vi "Event Start On Track.vi"(6 "Track ID":u64, 7 "Event Name":string, 8 "error in":errorcluster) -> (0 "error out":errorcluster)   [LabVIEW 2027, in "VS Tracing API.lvlib"]
doc: "Records the start of a user-space event on a previously registered custom track. The event remains active until the corresponding <i>Event Stop On Track</i> is called.\nUse this VI when recording events outside timed structures or when events need to be associated with a specific custom track.\n\n<b>Parameters</b>\n• <b>Track ID</b>: Identifier of the track created using <i>Register Track</i>.\n• <b>Event Name</b>: Name of the event to be displayed in the trace.\n\n<b>Notes</b>\n• Must be paired with <i>Event Stop On Track</i>.\n• The specified track must be registered before calling this VI."
uses:
  VS Tracing API.lvlib
  libvs_perfetto.dll
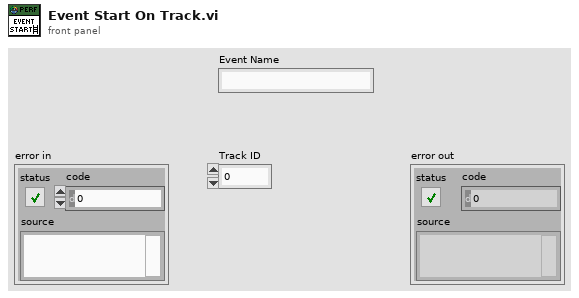
[diagram p1: front panel]
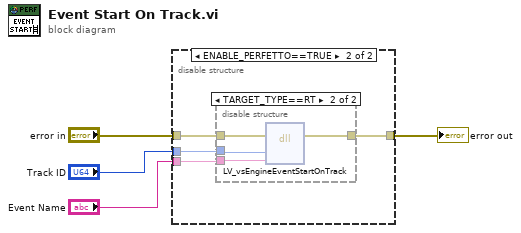
[diagram p0: block diagram]
diagram:
  n1 = disable-structure shown="ENABLE_PERFETTO==TRUE" {
    disable-tunnel: "Event Name" -> [_ w7]
    disable-tunnel: "error in" -> [w5 w8]
    disable-tunnel: [w5 w9] -> w3
    disable-tunnel: "Track ID" -> [_ w6]
    frame condition #0 (active) {
    }
    frame condition #1 {
      n2 = disable-structure shown="TARGET_TYPE==RT" {
        disable-tunnel: [w10 w14] -> w9
        disable-tunnel: w8 -> [w10 w13]
        disable-tunnel: w7 -> [_ w12]
        disable-tunnel: w6 -> [_ w11]
        frame condition #0 (active) {
        }
        frame condition #1 {
          n3 = dll-call lib="libvs_perfetto.*" fn="LV_vsEngineEventStartOnTrack"(error in=w13, "trackId"=w11, "eventName"=w12) -> (error out=w14:errorcluster)  [unwired: 5 in, 1 out]
        }
      }
    }
  }
  "error out" <- w3
